vi "Filtre ecg.vi"(3 "frequence echantillonage":dbl, 4 "Paramètre de filtrage":T1={"fréquence de coupure haute passe bande"=100.0, "fréquence de coupure basse passe bande"=0.3, "fréquence  de coupure haute stopbande"=52.0, "fréquence de coupure basse stopbande"=49.0, "ordre"=4, "passebande ON"=TRUE, "stopbande ON 2"=TRUE}, 5 "ECG":dbl[][](array[numeric])) -> (2 "ECG filtré":dbl[][](array[numeric]))   [LabVIEW 2017]
uses:
  <vilib>/Analysis/3filter.llb/Filter Passband Type.ctl
  <vilib>/Analysis/3filter.llb/Butterworth Filter (DBL).vi
  <vilib>/Analysis/NI_AALBase.lvlib
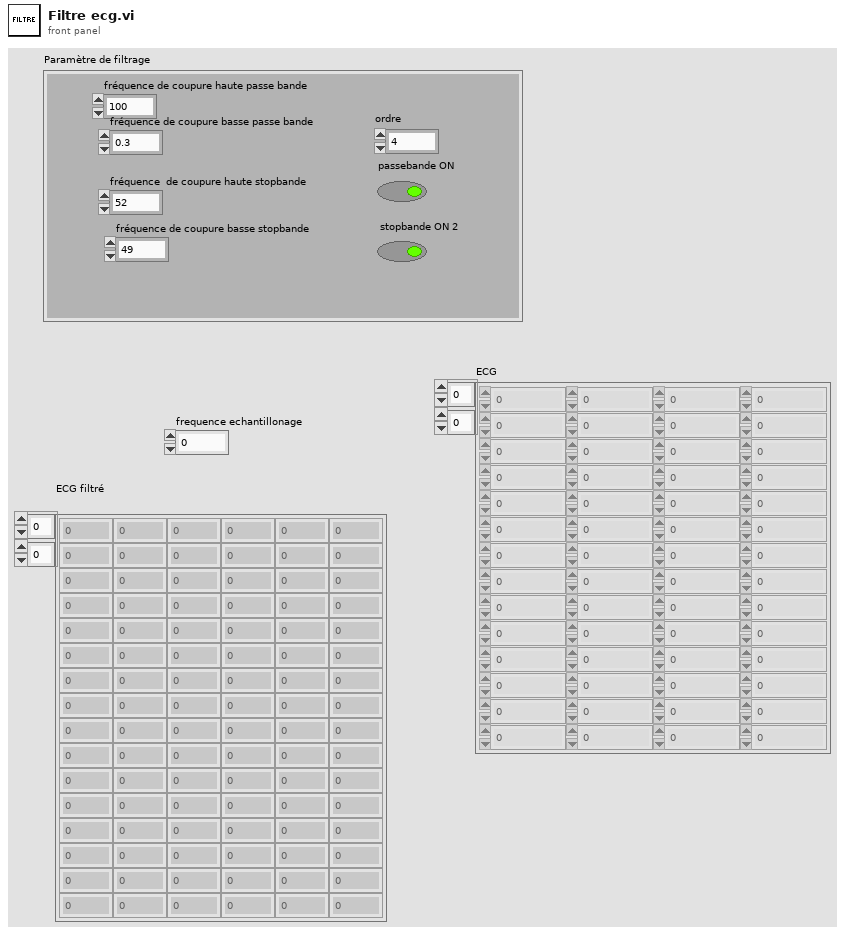
[diagram p1: front panel]
types:
  T1 = cluster{"fréquence de coupure haute passe bande":dbl, "fréquence de coupure basse passe bande":dbl, "fréquence  de coupure haute stopbande":dbl, "fréquence de coupure basse stopbande":dbl, "ordre":i32, "passebande ON":bool, "stopbande ON 2":bool}
  T2 = typedef "NI_AALBase.lvlib/Filter Passband Type.ctl" = enum32{"Lowpass", "Highpass", "Bandpass", "Bandstop"}
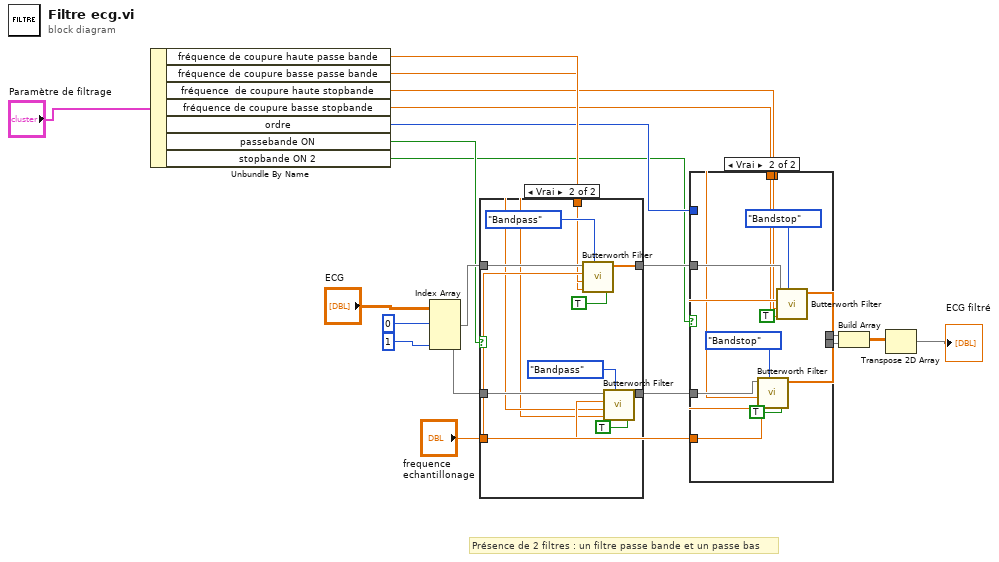
[diagram p0: block diagram]
diagram:
  # "Présence de 2 filtres : un filtre passe bande et un passe bas"
  n1 = Unbundle By Name("Paramètre de filtrage") -> ("fréquence de coupure haute passe bande"=w10:dbl, "fréquence de coupure basse passe bande"=w9:dbl, "fréquence  de coupure haute stopbande"=w8:dbl, "fréquence de coupure basse stopbande"=w7:dbl, "ordre"=w6:i32, "passebande ON"=w5:bool, "stopbande ON 2"=w4:bool)
  n2 = Index Array(array="ECG", index (col) #1=0 ("indice désactivé (col)"), index (col) #2=1 ("indice désactivé (col)")) -> (element #1=w12:dbl[], element #2=w11:dbl[])  [unwired: 2 in]
  n3 = case shown="Vrai" w5 {
    tunnel: [w21 w32] -> w15
    tunnel: [w22 w31] -> w14
    tunnel: "frequence echantillonage" -> [_ w30]
    tunnel: w12 -> [w22 w29]
    tunnel: w11 -> [w21 w28]
    tunnel: w10 -> [_ w26]
    tunnel: w9 -> [_ w25]
    frame False {
    }
    frame True {
      n4 = call-poly <vilib>:"Butterworth Filter.vi"("init/cont (init:F)"=TRUE, "filter type"=Filter_Passband_Type."Bandpass", "low cutoff freq: fl"=w25, "high cutoff freq: fh"=w26, "sampling freq: fs"=w30, "X"=w29) -> ("Filtered X"=w31:dbl[])  [unwired: 2 in, 1 out]
      n5 = call-poly <vilib>:"Butterworth Filter.vi"("init/cont (init:F)"=TRUE, "filter type"=Filter_Passband_Type."Bandpass", "low cutoff freq: fl"=w25, "high cutoff freq: fh"=w26, "sampling freq: fs"=w30, "X"=w28) -> ("Filtered X"=w32:dbl[])  [unwired: 2 in, 1 out]
    }
  }
  n6 = case shown="Vrai" w4 {
    tunnel: [w35 w46] -> w19
    tunnel: [w34 w45] -> w18
    tunnel: w15 -> [w34 w42]
    tunnel: w14 -> [w35 w41]
    tunnel: "frequence echantillonage" -> [_ w40]
    tunnel: w8 -> [_ w39]
    tunnel: w7 -> [_ w38]
    tunnel: w6 -> [_ _]
    frame False {
    }
    frame True {
      n7 = call-poly <vilib>:"Butterworth Filter.vi"("init/cont (init:F)"=TRUE, "filter type"=Filter_Passband_Type."Bandstop", "low cutoff freq: fl"=w38, "high cutoff freq: fh"=w39, "sampling freq: fs"=w40, "X"=w42) -> ("Filtered X"=w45:dbl[])  [unwired: 2 in, 1 out]
      n8 = call-poly <vilib>:"Butterworth Filter.vi"("init/cont (init:F)"=TRUE, "filter type"=Filter_Passband_Type."Bandstop", "low cutoff freq: fl"=w38, "high cutoff freq: fh"=w39, "sampling freq: fs"=w40, "X"=w41) -> ("Filtered X"=w46:dbl[])  [unwired: 2 in, 1 out]
    }
  }
  n9 = Build Array(w19, w18) -> (w17:dbl[][])
  n10 = Transpose 2D Array(2D array=w17) -> (transposed array=→"ECG filtré":dbl[][])
